vi "1B_BuildTriggerArray_LowCurrent.vi"(0 "CBC Trigger Level":dbl, 1 "Load Resistance (Ohms)":dbl, 2 "Target Stim Current (Amps)":dbl, 3 "Krec Value":i32, 4 "Recovery Mode (T=Active)":bool) -> (5 "Pulse Triggers":T1(array[cluster]))   [LabVIEW 2010]
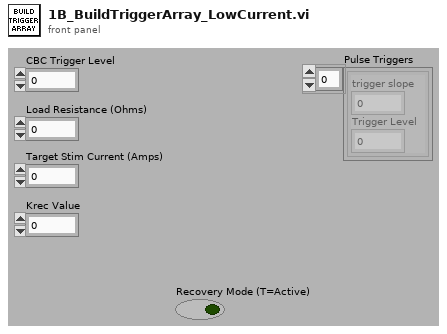
[diagram p1: front panel]
types:
  T1 = cluster{"trigger slope":u16, "Trigger Level":dbl}[]
  T2 = cluster{"trigger slope":u16, "Trigger Level":dbl}
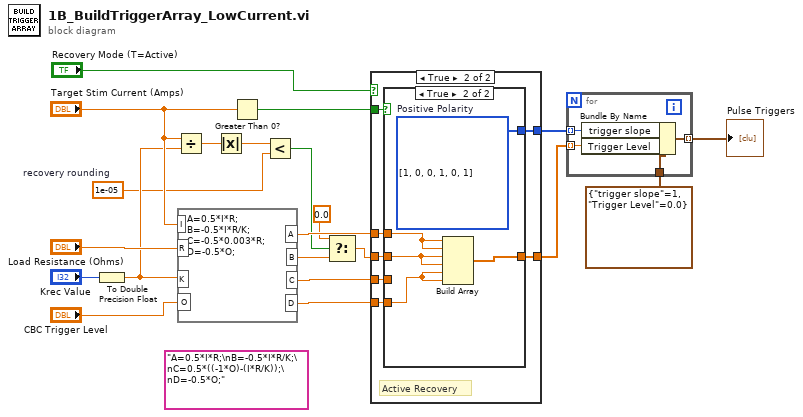
[diagram p0: block diagram]
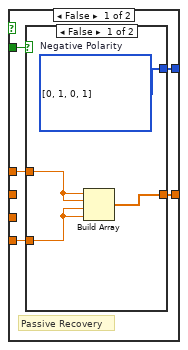
[diagram p2: hidden frame]
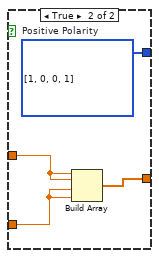
[diagram p3: hidden frame]
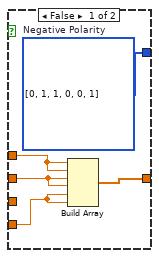
[diagram p4: hidden frame]
diagram:
  w6 = 1e-05  # recovery rounding
  (unwired) "A=0.5*I*R;\nB=-0.5*I*R/K;\nC=0.5*((-1*O)-(I*R/K));\nD=-0.5*O;"
  n1 = To Double Precision Float(number="Krec Value") -> (double precision float=w8:dbl)
  n2 = Divide(x="Target Stim Current (Amps)", y=w8) -> (x/y=w7:dbl)
  n3 = formula code="A=0.5*I*R;\nB=-0.5*I*R/K;\nC=-0.5*0.003*R;\nD=-0.5*O;"("R"="Load Resistance (Ohms)", "I"="Target Stim Current (Amps)", "K"=w8, "O"="CBC Trigger Level") -> ("A"=w13:dbl, "B"=w4:dbl, "C"=w12:dbl, "D"=w11:dbl)
  n4 = Absolute Value(x=w7) -> (abs(x)=w1:dbl)
  n5 = Greater Than 0?(x="Target Stim Current (Amps)") -> (x > 0?=w20:bool)
  n6 = Less?(x=w1, y=w6) -> (x < y?=w5:bool)
  n7 = Select(t=0.0, s=w5, f=w4) -> (s? t:f=w3:dbl)
  n8 = case shown="True" "Recovery Mode (T=Active)" {
    tunnel: [w25 w41] -> w17
    tunnel: w20 -> [w26 w40]
    tunnel: w13 -> [w24 w39]
    tunnel: w3 -> [_ w38]
    tunnel: w12 -> [_ w37]
    tunnel: w11 -> [w23 w36]
    tunnel: [w22 w35] -> w10
    frame False {
      # "Passive Recovery"
      n9 = case shown="False" w26 {
        tunnel: [w30 w34] -> w25
        tunnel: w24 -> [w29 w33]
        tunnel: w23 -> [w28 w32]
        tunnel: [w27 w31] -> w22
        frame False {
          w30 = u16[] [0, 1, 0, 1] items=["Falling Edge", "Rising Edge"]  # Negative Polarity
          n10 = Build Array(w29, w29, w28, w28) -> (w27:dbl[])
        }
        frame True {
          w34 = u16[] [1, 0, 0, 1] items=["Falling Edge", "Rising Edge"]  # Positive Polarity
          n11 = Build Array(w33, w33, w32, w32) -> (w31:dbl[])
        }
      }
    }
    frame True {
      # "Active Recovery"
      n12 = case shown="True" w40 {
        tunnel: [w46 w51] -> w41
        tunnel: w39 -> [w45 w50]
        tunnel: w38 -> [w43 w48]
        tunnel: w37 -> [_ _]
        tunnel: w36 -> [w42 w47]
        tunnel: [w44 w49] -> w35
        frame False {
          w46 = u16[] [0, 1, 1, 0, 0, 1] items=["Falling Edge", "Rising Edge"]  # Negative Polarity
          n13 = Build Array(w45, w45, w43, w43, w42, w42) -> (w44:dbl[])
        }
        frame True {
          w51 = u16[] [1, 0, 0, 1, 0, 1] items=["Falling Edge", "Rising Edge"]  # Positive Polarity
          n14 = Build Array(w50, w50, w48, w48, w47, w47) -> (w49:dbl[])
        }
      }
    }
  }
  n15 = for {
    tunnel: T2 {"trigger slope"=1, "Trigger Level"=0.0} -> [w55]
    tunnel: w17 -> [w54] mode=indexing
    tunnel: w10 -> [w53] mode=indexing
    tunnel: [w52] -> w19 mode=indexing
    n16 = Bundle By Name(cluster=w55, "trigger slope"=w54, "Trigger Level"=w53) -> (w52:T2)
  }
  "Pulse Triggers" <- w19
